vi "Drive.vi"(9 "CHASSIS":T6 {"vOmega" format="%10.3f"; "vY" format="%10.3f"; "vX" format="%10.3f"}, 11 "SWERVE_DRIVE_KINEMATICS":T1 {"SavedModuleStates"."Angle"."SIN" format="%13.4f"; "SavedModuleStates"."Angle"."COS" format="%13.4f"; "SavedModuleStates"."Angle"."VALUE" format="%13.4f"; "PrevCoR"."Y" format="%14.3f"; "PrevCoR"."X" format="%14.3f"; "Modules"."Y" format="%14.3f"; "Modules"."X" format="%14.3f"}) -> (1 "out WheelStates":T4[](array[typedef]) {"Angle"."SIN" format="%13.4f"; "Angle"."COS" format="%13.4f"; "Angle"."VALUE" format="%13.4f"}, 3 "out SWERVE_DRIVE_KINEMATICS":T1 {"SavedModuleStates"."Angle"."SIN" format="%13.4f"; "SavedModuleStates"."Angle"."COS" format="%13.4f"; "SavedModuleStates"."Angle"."VALUE" format="%13.4f"; "PrevCoR"."Y" format="%14.3f"; "PrevCoR"."X" format="%14.3f"; "Modules"."Y" format="%14.3f"; "Modules"."X" format="%14.3f"})   [LabVIEW 2023]
uses:
  <vilib>/Rock Robotics/WPI/ThirdParty/JAS_Junk/TrajLib/TypeDef/SWERVE_DRIVE_KINEMATICS.ctl
  <vilib>/Analysis/Matrix/Datatypes/RealMatrix.ctl
  <vilib>/Rock Robotics/WPI/ThirdParty/JAS_Junk/TrajLib/TypeDef/TRANSLATION2D.ctl
  <vilib>/Rock Robotics/WPI/ThirdParty/JAS_Junk/TrajLib/TypeDef/SWERVE_DRIVE_MODULE_STATE.ctl
  <vilib>/Rock Robotics/WPI/ThirdParty/JAS_Junk/TrajLib/TypeDef/ROTATION2D.ctl
  <vilib>/Rock Robotics/WPI/ThirdParty/JAS_Junk/TrajLib/TypeDef/CHASSIS_SPEEDS.ctl
  <vilib>/Rock Robotics/WPI/ThirdParty/REV Robotics/REVLib/Typedef/Spark MAX Control Type.ctl
  <vilib>/Rock Robotics/WPI/ThirdParty/JAS_Junk/TrajLib/Rotation2d_Minus.vi
  <vilib>/Rock Robotics/WPI/ThirdParty/JAS_Junk/TrajLib/Rotation2d_GetRadians.vi
  <vilib>/Rock Robotics/WPI/ThirdParty/JAS_Junk/TrajLib/SwerveModuleState_New.vi
  <vilib>/Rock Robotics/WPI/ThirdParty/JAS_Junk/TrajLib/Rotation2d_RotateBy.vi
  <vilib>/Rock Robotics/WPI/ThirdParty/JAS_Junk/TrajLib/Rotation2d_UnaryMinus.vi
  <vilib>/Rock Robotics/WPI/ThirdParty/JAS_Junk/TrajLib/Rotation2d_CreateXY.vi
  <vilib>/Rock Robotics/WPI/ThirdParty/JAS_Junk/TrajLib/Util_CalcDist.vi
  <vilib>/Analysis/Matrix/Comparison/Equal/Equal.vi
  <vilib>/Analysis/Matrix/Comparison/Equal/Equal - RM,RM.vi
  <vilib>/Utility/AggHandler/Cls_AggHandler.xnode
  <vilib>/Rock Robotics/WPI/ThirdParty/JAS_Junk/TrajLib/Trajectory_Library.lvlib
  <vilib>/Analysis/Matrix/NI_Matrix.lvlib
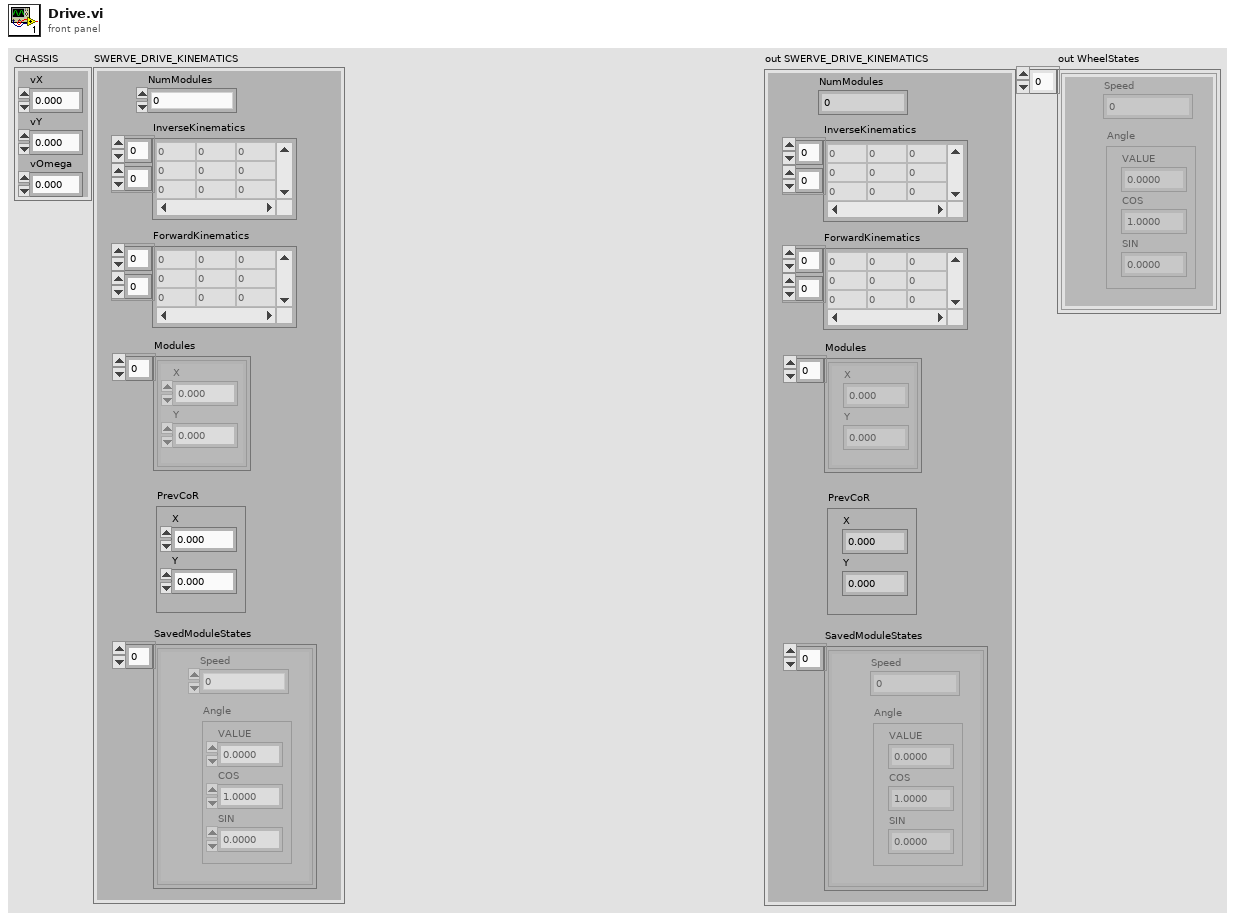
[diagram p1: front panel]
types:
  T1 = typedef "Trajectory_Library.lvlib/SWERVE_DRIVE_KINEMATICS.ctl" = cluster{"NumModules":i32, "InverseKinematics":T2, "ForwardKinematics":T2, "Modules":T3[], "PrevCoR":T3, "SavedModuleStates":T4[]}
  T2 = typedef "NI_Matrix.lvlib/RealMatrix.ctl" = dbl[][]
  T3 = typedef "Trajectory_Library.lvlib/TRANSLATION2D.ctl" = cluster{"X":dbl, "Y":dbl}
  T4 = typedef "Trajectory_Library.lvlib/SWERVE_DRIVE_MODULE_STATE.ctl" = cluster{"Speed":dbl, "Angle":T5}
  T5 = typedef "Trajectory_Library.lvlib/ROTATION2D.ctl" = cluster{"VALUE":dbl, "COS":dbl, "SIN":dbl}
  T6 = typedef "Trajectory_Library.lvlib/CHASSIS_SPEEDS.ctl" = cluster{"vX":dbl, "vY":dbl, "vOmega":dbl}
  T7 = typedef "WPI_MotorControlDeviceRef.ctl" = cluster{"DeviceStatus":errorcluster, "Type":T8, "PWM":cluster{"PWM Channel":T9, "DeadBand":T10}, "CAN":cluster{"Device Number":u8, "SetOutput VI Ref":variant, "GetOutput VI Ref":variant, "Enable VI Ref":variant, "Disable VI Ref":variant, "Data":variant}, "Invert":bool, "DIO PWM":cluster{"PWM \"Enable\" Channel":T9, "DIOChannel":T11, "PWM Rate":dbl}}
  T8 = typedef "WPI_MotorControlType.ctl" = enum16{"PWM", "CAN", "DIO PWM"}
  T9 = typedef "FPGA_DIOPWMChannel.ctl" = enum8{"PWM 0", "PWM 1", "PWM 2", "PWM 3", "PWM 4", "PWM 5", "PWM 6", "PWM 7", "PWM 8", "PWM 9", "PWM MXP 0", "PWM MXP 1", "PWM MXP 2", "PWM MXP 3", "PWM MXP 4", "PWM MXP 5", "PWM MXP 6", "PWM MXP 7", "PWM MXP 8", "PWM MXP 9", "Invalid"}
  T10 = typedef "WPI_PWMDeadband.ctl" = cluster{"Name":string, "maxPositivePwm":i32, "minPositivePwm":i32, "centerPwm":i32, "maxNegativePwm":i32, "minNegativePwm":i32, "angularRange":u16}
  T11 = typedef "FPGA_DIOChannel.ctl" = enum8{"DIO 0", "DIO 1", "DIO 2", "DIO 3", "DIO 4", "DIO 5", "DIO 6", "DIO 7", "DIO 8", "DIO 9", "DIO MXP 0", "DIO MXP 1", "DIO MXP 2", "DIO MXP 3", "DIO MXP 4", "DIO MXP 5", "DIO MXP 6", "DIO MXP 7", "DIO MXP 8", "DIO MXP 9", "DIO MXP 10", "DIO MXP 11", "DIO MXP 12", "DIO MXP 13", "DIO MXP 14", "DIO MXP 15", "SPI Port CS1", "SPI Port CS2", "SPI Port CS3", "SPI Port MISO", "SPI Port MOSI", "Invalid"}
  T12 = typedef "Spark MAX Control Type.ctl" = enum16{"Percent VBus", "Voltage", "Velocity", "Position", "Smart Motion", "Current", "Smart Velocity"}
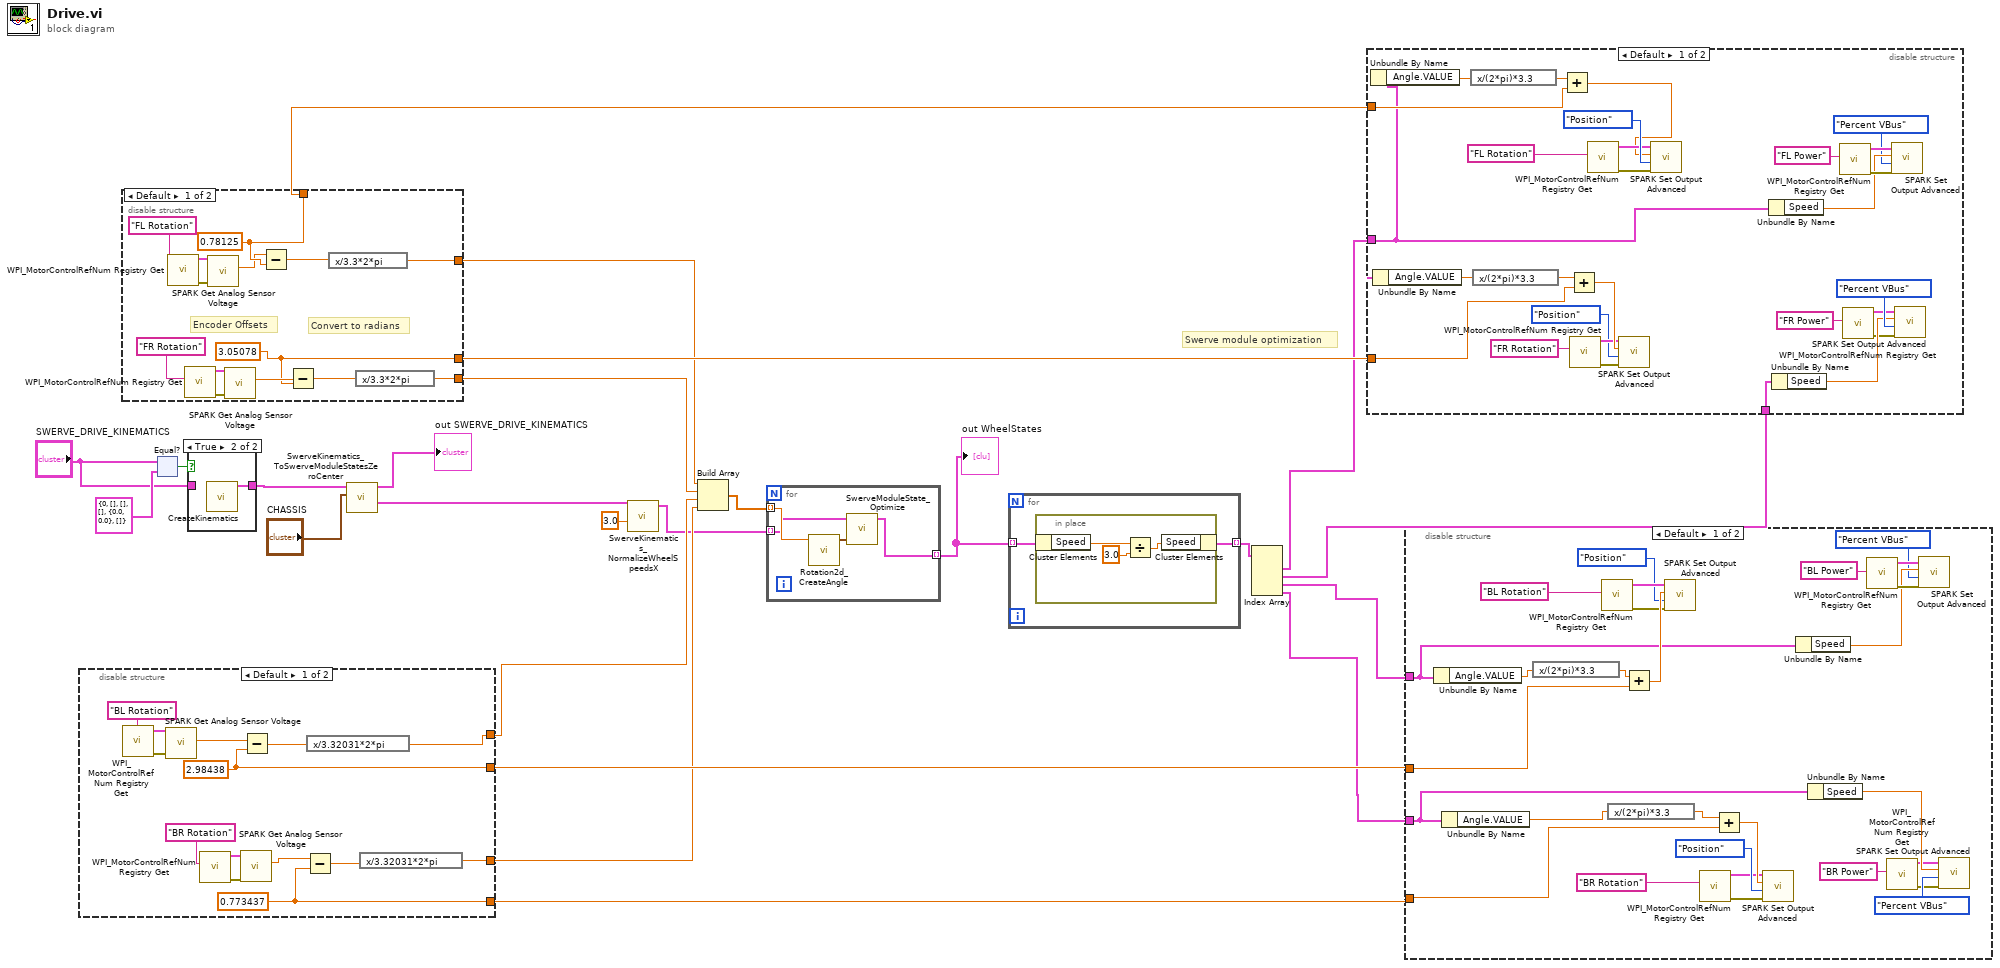
[diagram p0: block diagram]
diagram:
  # "Swerve module optimization"
  n1 = disable-structure shown="Default" {
    disable-tunnel: [w38 _] -> w24
    disable-tunnel: [w29 _] -> w18
    disable-tunnel: [w27 _] -> w20
    disable-tunnel: [w25 _] -> w19
    frame condition #0 (active) {
      w27 = 0.773437 ("x")
      w38 = 2.98438 ("y")
      n2 = call <vilib>:"WPI_MotorControlRefNum Registry Get.vi"("refnum name"="BL Rotation") -> ("error out"=w32:errorcluster, "MotorControlDevRef"=w33:T7)  [unwired: 9 in]
      n3 = call <vilib>:"SPARK Get Analog Sensor Voltage.vi"("error in (no error)"=w32, "MotorControlDevRef in"=w33) -> ("Analog Sensor Voltage"=w37:dbl)  [unwired: 6 in, 3 out]
      n4 = call <vilib>:"WPI_MotorControlRefNum Registry Get.vi"("refnum name"="BR Rotation") -> ("error out"=w35:errorcluster, "MotorControlDevRef"=w34:T7)  [unwired: 9 in]
      n5 = call <vilib>:"SPARK Get Analog Sensor Voltage.vi"("error in (no error)"=w35, "MotorControlDevRef in"=w34) -> ("Analog Sensor Voltage"=w28:dbl)  [unwired: 6 in, 3 out]
      n6 = Subtract(x=w37, y=w38) -> (x-y=w30:dbl)
      n7 = Subtract(x=w28, y=w27) -> (x-y=w26:dbl)
      n8 = expression code="x/3.32031*2*pi"(w30) -> (w29:dbl)
      n9 = expression code="x/3.32031*2*pi"(w26) -> (w25:dbl)
    }
    frame condition #1 {
    }
  }
  n10 = disable-structure shown="Default" {
    disable-tunnel: [w52 _] -> w22
    disable-tunnel: [w43 _] -> w16
    disable-tunnel: [w41 _] -> w21
    disable-tunnel: [w39 _] -> w17
    frame condition #0 (active) {
      w41 = 3.05078 ("y")
      w52 = 0.78125 ("y")
      # "Convert to radians"
      # "Encoder Offsets"
      n11 = call <vilib>:"WPI_MotorControlRefNum Registry Get.vi"("refnum name"="FL Rotation") -> ("error out"=w47:errorcluster, "MotorControlDevRef"=w48:T7)  [unwired: 9 in]
      n12 = call <vilib>:"WPI_MotorControlRefNum Registry Get.vi"("refnum name"="FR Rotation") -> ("error out"=w50:errorcluster, "MotorControlDevRef"=w49:T7)  [unwired: 9 in]
      n13 = call <vilib>:"SPARK Get Analog Sensor Voltage.vi"("error in (no error)"=w47, "MotorControlDevRef in"=w48) -> ("Analog Sensor Voltage"=w45:dbl)  [unwired: 6 in, 3 out]
      n14 = call <vilib>:"SPARK Get Analog Sensor Voltage.vi"("error in (no error)"=w50, "MotorControlDevRef in"=w49) -> ("Analog Sensor Voltage"=w42:dbl)  [unwired: 6 in, 3 out]
      n15 = Subtract(x=w45, y=w52) -> (x-y=w44:dbl)
      n16 = Subtract(x=w42, y=w41) -> (x-y=w40:dbl)
      n17 = expression code="x/3.3*2*pi"(w44) -> (w43:dbl)
      n18 = expression code="x/3.3*2*pi"(w40) -> (w39:dbl)
    }
    frame condition #1 {
    }
  }
  n19 = xnode "Equal?"("Y"=T1 {"NumModules"=0, "InverseKinematics"=[], "ForwardKinematics"=[], "Modules"=[], "PrevCoR"={"X"=0.0, "Y"=0.0}, "SavedModuleStates"=[]} ("SWERVE_DRIVE_KINEMATICS 2"), "X"="SWERVE_DRIVE_KINEMATICS") -> ("Z"=w3:bool)
  n20 = case shown="True" w3 {
    tunnel: [w53 w54] -> w4
    tunnel: "SWERVE_DRIVE_KINEMATICS" -> [w53 _]
    frame False {
    }
    frame True {
      n21 = call "CreateKinematics.vi"() -> ("SWERVE_DRIVE_KINEMATICS"=w54:T1)  [unwired: 11 in]
    }
  }
  n22 = call <vilib>:"SwerveKinematics_ToSwerveModuleStatesZeroCenter.vi"("ChassisSpeeds"="CHASSIS", "in SWERVE_DRIVE_KINEMATICS"=w4) -> ("ModuleStates"=w5:T4[], "out SWERVE_DRIVE_KINEMATICS"=→"out SWERVE_DRIVE_KINEMATICS":T1)  [unwired: 8 in]
  n23 = call <vilib>:"SwerveKinematics_NormalizeWheelSpeedsX.vi"("AttainableMaxSpeed"=3.0, "in WheelStates"=w5) -> ("out WheelStates"=w14:T4[])  [unwired: 9 in]
  n24 = Build Array(w16, w17, w18, w19) -> (w15:dbl[])
  n25 = for {
    tunnel: w15 -> [w58] mode=indexing
    tunnel: w14 -> [w56] mode=indexing
    tunnel: [w55] -> w9 mode=indexing
    n26 = call <vilib>:"Rotation2d_CreateAngle.vi"("Angle"=w58) -> ("ROTATION"=w57:T5)  [unwired: 10 in]
    n27 = call <vilib>:"SwerveModuleState_Optimize.vi"("CurrentAngle"=w57, "Desired State"=w56) -> ("out SWERVE_DRIVE_MODULE_STATE"=w55:T4)  [unwired: 9 in]
  }
  "out WheelStates" <- w9
  n28 = for {
    tunnel: w9 -> [w60] mode=indexing
    tunnel: [w59] -> w8 mode=indexing
    n29 = in-place {
      n30 = in-place-cluster #1(w60) -> ("Speed"=w63:dbl)
      n31 = Divide(x=w63, y=3.0) -> (x/y=w61:dbl)
      n32 = in-place-cluster #1("Speed"=w61) -> (w59:T4)
    }
  }
  n33 = Index Array(array=w8) -> (element #1=w13:T4, element #2=w12:T4, element #3=w11:T4, element #4=w10:T4)  [unwired: 4 in]
  n34 = disable-structure shown="Default" {
    disable-tunnel: w21 -> [w70 _]
    disable-tunnel: w12 -> [w69 _]
    disable-tunnel: w13 -> [w65 _]
    disable-tunnel: w22 -> [w66 _]
    frame condition #0 (active) {
      n35 = Unbundle By Name(w65) -> ("Angle.VALUE"=w67:dbl)
      n36 = Unbundle By Name(w69) -> ("Angle.VALUE"=w89:dbl)
      n37 = expression code="x/(2*pi)*3.3"(w67) -> (w68:dbl)
      n38 = expression code="x/(2*pi)*3.3"(w89) -> (w90:dbl)
      n39 = Add(x=w68, y=w66) -> (x+y=w64:dbl)
      n40 = Add(x=w90, y=w70) -> (x+y=w91:dbl)
      n41 = call <vilib>:"WPI_MotorControlRefNum Registry Get.vi"("refnum name"="FR Rotation") -> ("error out"=w77:errorcluster, "MotorControlDevRef"=w76:T7)  [unwired: 9 in]
      n42 = call <vilib>:"WPI_MotorControlRefNum Registry Get.vi"("refnum name"="FL Rotation") -> ("error out"=w72:errorcluster, "MotorControlDevRef"=w73:T7)  [unwired: 9 in]
      n43 = call <vilib>:"SPARK Set Output Advanced.vi"("error in (no error)"=w77, "Control Mode"=Spark_MAX_Control_Type."Position", "Setpoint"=w91, "MotorControlDevRef"=w76) -> ()  [unwired: 6 in, 2 out]
      n44 = call <vilib>:"SPARK Set Output Advanced.vi"("error in (no error)"=w72, "Control Mode"=Spark_MAX_Control_Type."Position", "Setpoint"=w64, "MotorControlDevRef"=w73) -> ()  [unwired: 6 in, 2 out]
      n45 = Unbundle By Name(w65) -> ("Speed"=w81:dbl)
      n46 = Unbundle By Name(w69) -> ("Speed"=w86:dbl)
      n47 = call <vilib>:"WPI_MotorControlRefNum Registry Get.vi"("refnum name"="FL Power") -> ("error out"=w83:errorcluster, "MotorControlDevRef"=w82:T7)  [unwired: 9 in]
      n48 = call <vilib>:"WPI_MotorControlRefNum Registry Get.vi"("refnum name"="FR Power") -> ("error out"=w84:errorcluster, "MotorControlDevRef"=w85:T7)  [unwired: 9 in]
      n49 = call <vilib>:"SPARK Set Output Advanced.vi"("error in (no error)"=w83, "Control Mode"=Spark_MAX_Control_Type."Percent VBus", "Setpoint"=w81, "MotorControlDevRef"=w82) -> ()  [unwired: 6 in, 2 out]
      n50 = call <vilib>:"SPARK Set Output Advanced.vi"("error in (no error)"=w84, "Control Mode"=Spark_MAX_Control_Type."Percent VBus", "Setpoint"=w86, "MotorControlDevRef"=w85) -> ()  [unwired: 6 in, 2 out]
    }
    frame condition #1 {
    }
  }
  n51 = disable-structure shown="Default" {
    disable-tunnel: w10 -> [w112 _]
    disable-tunnel: w11 -> [w111 _]
    disable-tunnel: w24 -> [w93 _]
    disable-tunnel: w20 -> [w92 _]
    frame condition #0 (active) {
      n52 = Unbundle By Name(w111) -> ("Angle.VALUE"=w114:dbl)
      n53 = Unbundle By Name(w112) -> ("Angle.VALUE"=w119:dbl)
      n54 = expression code="x/(2*pi)*3.3"(w114) -> (w115:dbl)
      n55 = call <vilib>:"WPI_MotorControlRefNum Registry Get.vi"("refnum name"="BL Rotation") -> ("error out"=w100:errorcluster, "MotorControlDevRef"=w99:T7)  [unwired: 9 in]
      n56 = expression code="x/(2*pi)*3.3"(w119) -> (w117:dbl)
      n57 = Add(x=w115, y=w93) -> (x+y=w116:dbl)
      n58 = call <vilib>:"SPARK Set Output Advanced.vi"("error in (no error)"=w100, "Control Mode"=Spark_MAX_Control_Type."Position", "Setpoint"=w116, "MotorControlDevRef"=w99) -> ()  [unwired: 6 in, 2 out]
      n59 = call <vilib>:"WPI_MotorControlRefNum Registry Get.vi"("refnum name"="BR Rotation") -> ("error out"=w95:errorcluster, "MotorControlDevRef"=w96:T7)  [unwired: 9 in]
      n60 = Add(x=w117, y=w92) -> (x+y=w118:dbl)
      n61 = call <vilib>:"SPARK Set Output Advanced.vi"("error in (no error)"=w95, "Control Mode"=Spark_MAX_Control_Type."Position", "Setpoint"=w118, "MotorControlDevRef"=w96) -> ()  [unwired: 6 in, 2 out]
      n62 = Unbundle By Name(w111) -> ("Speed"=w103:dbl)
      n63 = Unbundle By Name(w112) -> ("Speed"=w108:dbl)
      n64 = call <vilib>:"WPI_MotorControlRefNum Registry Get.vi"("refnum name"="BL Power") -> ("error out"=w105:errorcluster, "MotorControlDevRef"=w104:T7)  [unwired: 9 in]
      n65 = call <vilib>:"WPI_MotorControlRefNum Registry Get.vi"("refnum name"="BR Power") -> ("error out"=w106:errorcluster, "MotorControlDevRef"=w107:T7)  [unwired: 9 in]
      n66 = call <vilib>:"SPARK Set Output Advanced.vi"("error in (no error)"=w105, "Control Mode"=Spark_MAX_Control_Type."Percent VBus", "Setpoint"=w103, "MotorControlDevRef"=w104) -> ()  [unwired: 6 in, 2 out]
      n67 = call <vilib>:"SPARK Set Output Advanced.vi"("error in (no error)"=w106, "Control Mode"=Spark_MAX_Control_Type."Percent VBus", "Setpoint"=w108, "MotorControlDevRef"=w107) -> ()  [unwired: 6 in, 2 out]
    }
    frame condition #1 {
    }
  }
